vi "activateDoorMotionActivationSignals.vi"(7 "Door Context:":T1, 8 "error in (no error)":errorcluster, 9 "activateOpenMotionIsT":bool, 10 "activateCloseMotionIsT":bool, 11 "cRIOScanModeTarget in":refnum<class "cRIOScanModeTarget.lvclass">) -> (0 "error out":errorcluster, 3 "cRIOScanModeTarget out":refnum<class "cRIOScanModeTarget.lvclass">)   [LabVIEW 2012, in "cRIOScanModeTarget.lvclass"]
doc: "Sends the specified values to the activate close and open motion signals to the specified door."
uses:
  cRIOScanModeTarget.lvclass
  VentilationDoor/Typedefs/DoorContext.ctl
  VentilationDoor/Typedefs/VCDVentilationDoorTypedefs.lvlib
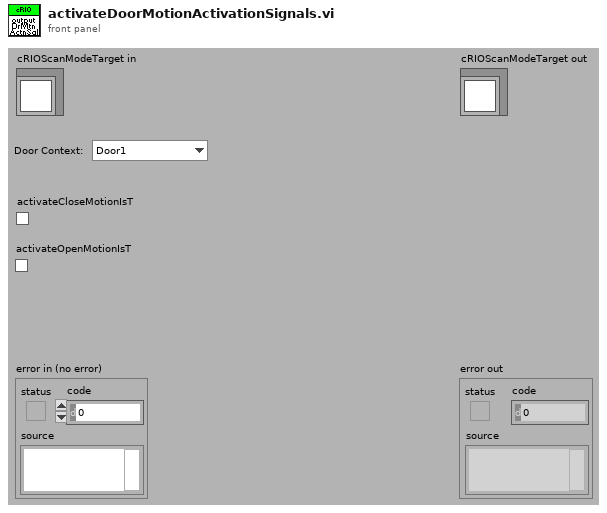
[diagram p1: front panel]
types:
  T1 = typedef "VCDVentilationDoorTypedefs.lvlib/DoorContext.ctl" = enum16{"Door1", "Door2", "Door3", "Door4", "Door5", "Door6", "Door7"}
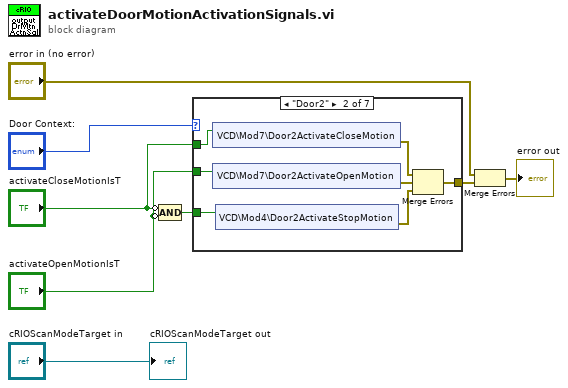
[diagram p0: block diagram]
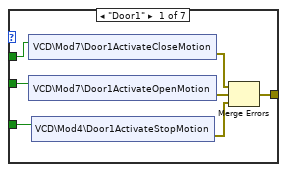
[diagram p2: hidden frame]
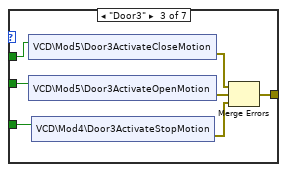
[diagram p3: hidden frame]
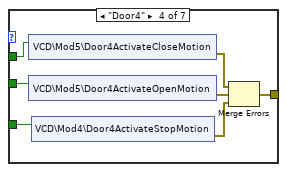
[diagram p4: hidden frame]
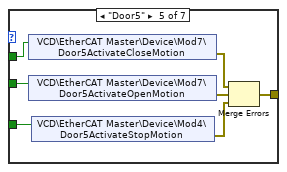
[diagram p5: hidden frame]
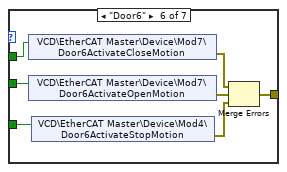
[diagram p6: hidden frame]
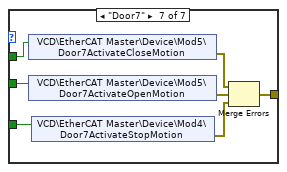
[diagram p7: hidden frame]
diagram:
  n1 = Compound Arithmetic op=AND(invert "activateCloseMotionIsT", invert "activateOpenMotionIsT") -> (w2:bool)
  n2 = case shown="\"Door2\"" "Door Context:" {
    tunnel: "activateCloseMotionIsT" -> [w11 w16 w25 w32 w39 w46 w53]
    tunnel: w2 -> [w9 w18 w23 w30 w37 w44 w51]
    tunnel: [w13 w19 w26 w33 w43 w50 w57] -> w3
    tunnel: "activateOpenMotionIsT" -> [w10 w17 w24 w31 w38 w45 w52]
    frame "Door1" {
      n3 = shared-variable "VCD\\Mod7\\Door1ActivateCloseMotion"(w11) -> (error out=w12:errorcluster)  [unwired: 1 in]
      n4 = shared-variable "VCD\\Mod7\\Door1ActivateOpenMotion"(w10) -> (error out=w15:errorcluster)  [unwired: 1 in]
      n5 = shared-variable "VCD\\Mod4\\Door1ActivateStopMotion"(w9) -> (error out=w14:errorcluster)  [unwired: 1 in]
      n6 = Merge Errors(w12, w15, w14) -> (w13:errorcluster)
    }
    frame "Door2" {
      n7 = shared-variable "VCD\\Mod7\\Door2ActivateCloseMotion"(w16) -> (error out=w22:errorcluster)  [unwired: 1 in]
      n8 = shared-variable "VCD\\Mod7\\Door2ActivateOpenMotion"(w17) -> (error out=w21:errorcluster)  [unwired: 1 in]
      n9 = shared-variable "VCD\\Mod4\\Door2ActivateStopMotion"(w18) -> (error out=w20:errorcluster)  [unwired: 1 in]
      n10 = Merge Errors(w22, w21, w20) -> (w19:errorcluster)
    }
    frame "Door3" {
      n11 = shared-variable "VCD\\Mod5\\Door3ActivateCloseMotion"(w25) -> (error out=w29:errorcluster)  [unwired: 1 in]
      n12 = shared-variable "VCD\\Mod5\\Door3ActivateOpenMotion"(w24) -> (error out=w28:errorcluster)  [unwired: 1 in]
      n13 = shared-variable "VCD\\Mod4\\Door3ActivateStopMotion"(w23) -> (error out=w27:errorcluster)  [unwired: 1 in]
      n14 = Merge Errors(w29, w28, w27) -> (w26:errorcluster)
    }
    frame "Door4" {
      n15 = shared-variable "VCD\\Mod5\\Door4ActivateCloseMotion"(w32) -> (error out=w36:errorcluster)  [unwired: 1 in]
      n16 = shared-variable "VCD\\Mod5\\Door4ActivateOpenMotion"(w31) -> (error out=w35:errorcluster)  [unwired: 1 in]
      n17 = shared-variable "VCD\\Mod4\\Door4ActivateStopMotion"(w30) -> (error out=w34:errorcluster)  [unwired: 1 in]
      n18 = Merge Errors(w36, w35, w34) -> (w33:errorcluster)
    }
    frame "Door5" {
      n19 = shared-variable "VCD\\EtherCAT Master\\Device\\Mod7\\Door5ActivateCloseMotion"(w39) -> (error out=w41:errorcluster)  [unwired: 1 in]
      n20 = shared-variable "VCD\\EtherCAT Master\\Device\\Mod7\\Door5ActivateOpenMotion"(w38) -> (error out=w42:errorcluster)  [unwired: 1 in]
      n21 = shared-variable "VCD\\EtherCAT Master\\Device\\Mod4\\Door5ActivateStopMotion"(w37) -> (error out=w40:errorcluster)  [unwired: 1 in]
      n22 = Merge Errors(w41, w42, w40) -> (w43:errorcluster)
    }
    frame "Door6" {
      n23 = shared-variable "VCD\\EtherCAT Master\\Device\\Mod7\\Door6ActivateCloseMotion"(w46) -> (error out=w48:errorcluster)  [unwired: 1 in]
      n24 = shared-variable "VCD\\EtherCAT Master\\Device\\Mod7\\Door6ActivateOpenMotion"(w45) -> (error out=w47:errorcluster)  [unwired: 1 in]
      n25 = shared-variable "VCD\\EtherCAT Master\\Device\\Mod4\\Door6ActivateStopMotion"(w44) -> (error out=w49:errorcluster)  [unwired: 1 in]
      n26 = Merge Errors(w48, w47, w49) -> (w50:errorcluster)
    }
    frame "Door7" {
      n27 = shared-variable "VCD\\EtherCAT Master\\Device\\Mod5\\Door7ActivateCloseMotion"(w53) -> (error out=w55:errorcluster)  [unwired: 1 in]
      n28 = shared-variable "VCD\\EtherCAT Master\\Device\\Mod5\\Door7ActivateOpenMotion"(w52) -> (error out=w54:errorcluster)  [unwired: 1 in]
      n29 = shared-variable "VCD\\EtherCAT Master\\Device\\Mod4\\Door7ActivateStopMotion"(w51) -> (error out=w56:errorcluster)  [unwired: 1 in]
      n30 = Merge Errors(w55, w54, w56) -> (w57:errorcluster)
    }
  }
  n31 = Merge Errors("error in (no error)", w3) -> (→"error out":errorcluster)
  "cRIOScanModeTarget out" <- "cRIOScanModeTarget in"
